vi "Update if Clear.vi"(8 "error in (no error)":errorcluster, 10 "Message Data":variant, 11 "Queue in":refnum<queue>) -> (0 "error out":errorcluster)   [LabVIEW 2018, in "Support Library.lvlib"]
uses:
  Support Library.lvlib
  Message Queue/Message Cluster.ctl
  Message Queue/Enqueue Message (Single).vi
  Message Queue/Message Queue.lvlib
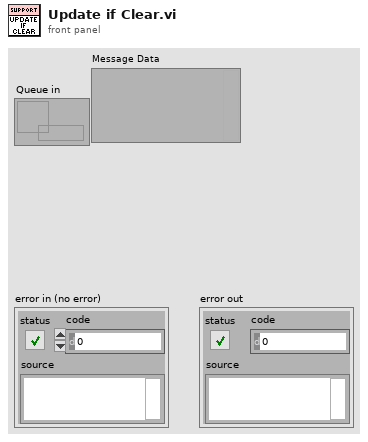
[diagram p1: front panel]
types:
  T1 = typedef "Support Library.lvlib/Message Queue.lvlib/Message Cluster.ctl" = cluster{"Message":string, "Message Data":variant}
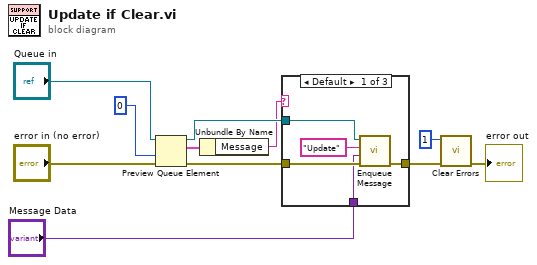
[diagram p0: block diagram]
diagram:
  n1 = Preview Queue Element(queue="Queue in", timeout in ms (-1)=0, error in (no error)="error in (no error)") -> (queue out=w8:refnum<queue>, element=w7:T1, error out=w5:errorcluster)  [unwired: 1 out]
  n2 = Unbundle By Name(w7) -> ("Message"=w6:string)
  n3 = case shown="Default" w6 {
    tunnel: w8 -> [w13 _ _]
    tunnel: [w14 w17 w18] -> w2
    tunnel: w5 -> [w15 w17 w18]
    tunnel: "Message Data" -> [w12 _ _]
    frame Default {
      n4 = call-poly "Enqueue Message.vi"("error in (no error)"=w15, "Message Data"=w12, "Message"="Update", "Message Queue"=w13) -> ("error out"=w14:errorcluster)  [unwired: 6 in, 1 out]
    }
    frame "Update" {
    }
    frame "Exit" {
    }
  }
  n5 = call <vilib>:"Clear Errors.vi"("error in (no error)"=w2, "specific error code to clear (0: all)"=1) -> ("error out"=→"error out":errorcluster)  [unwired: 4 in, 1 out]
